vi "FlatToRichcif_management_common_MonitorDoubles.vi"(5 "OutputClusterType":T1, 11 "InputCluster":T2) -> (3 "OutputCluster":T1)   [LabVIEW 2021, in "CIFCoreChannel_client.lvlib"]
uses:
  cif_management_common_MonitorDoubles_Flat.ctl
  cif_management_common_MonitorDoubles.ctl
  CIFCoreChannel_client.lvlib
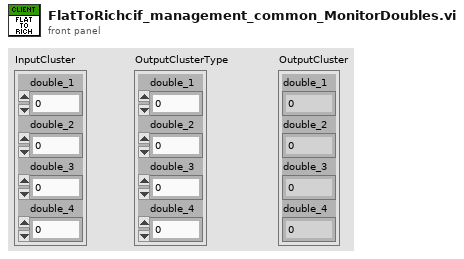
[diagram p1: front panel]
types:
  T1 = typedef "CIFCoreChannel_client.lvlib/cif_management_common_MonitorDoubles.ctl" = cluster{"double_1":dbl, "double_2":dbl, "double_3":dbl, "double_4":dbl}
  T2 = typedef "CIFCoreChannel_client.lvlib/cif_management_common_MonitorDoubles_Flat.ctl" = cluster{"double_1":dbl, "double_2":dbl, "double_3":dbl, "double_4":dbl}
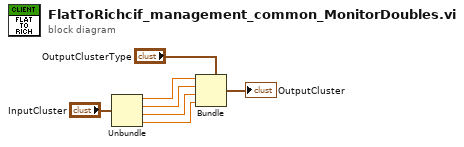
[diagram p0: block diagram]
diagram:
  n1 = Unbundle "Unbundle"("InputCluster") -> ("double_1"=w4:dbl, "double_2"=w3:dbl, "double_3"=w2:dbl, "double_4"=w1:dbl)
  n2 = Bundle "Bundle"(cluster="OutputClusterType", "double_1"=w4, "double_2"=w3, "double_3"=w2, "double_4"=w1) -> (→"OutputCluster":T1)
